vi "TDMS.SetMetadata.vi"(0 "Data":path, 2 "DUTs.AppVersion":string, 11 "error in (no error)":errorcluster, 13 "DUTs.BootVersion":string) -> (15 "error out":errorcluster)   [LabVIEW 2014, in "ParametericRoutines.lvlib"]
uses:
  ParametericRoutines.lvlib
  Constants.vi
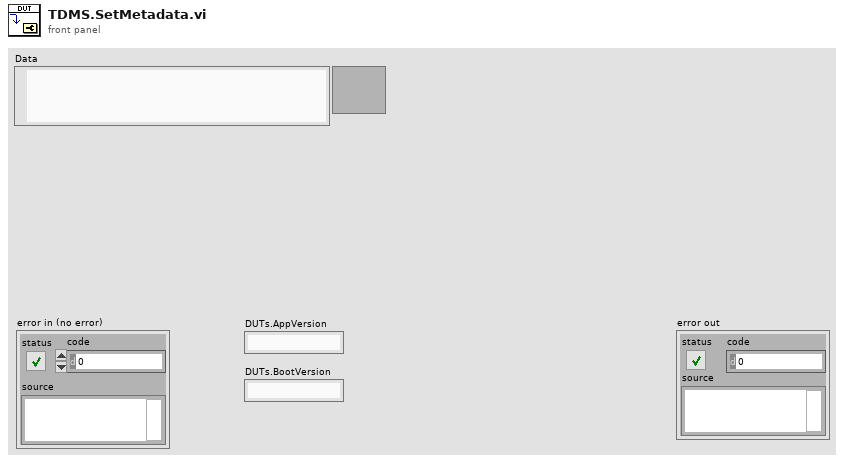
[diagram p1: front panel]
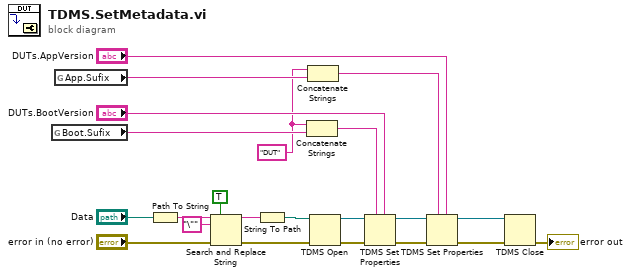
[diagram p0: block diagram]
diagram:
  w3 = "DUT" ("Boot.Sufix")
  n1 = global read "Constants.vi" "Boot.Sufix"() -> (w13:string)
  n2 = global read "Constants.vi" "App.Sufix"() -> (w14:string)
  n3 = Path To String(path="Data") -> (string=w21:string)
  n4 = Search and Replace String(replace all?=TRUE ("replace all? (F)"), input string=w21, search string="\"", error in="error in (no error)") -> (result string=w22:string, error out=w16:errorcluster)  [unwired: 4 in, 2 out]
  n5 = String To Path(string=w22) -> (path=w17:path)
  n6 = Concatenate Strings(w3, w13) -> (w7:string)
  n7 = Concatenate Strings(w3, w14) -> (w6:string)
  n8 = TDMS Open(8:w16, 11:w17) -> (0:w1:errorcluster, 3:w2:refnum<k34>)  [unwired: 5 in]
  n9 = TDMS Set Properties(5:"DUTs.BootVersion", 7:w7, 8:w1, 11:w2) -> (0:w8:errorcluster, 3:w9:refnum<k34>)  [unwired: 2 in, 2 out]
  n10 = TDMS Set Properties(5:"DUTs.AppVersion", 7:w6, 8:w8, 11:w9) -> (0:w12:errorcluster, 3:w11:refnum<k34>)  [unwired: 2 in, 2 out]
  n11 = TDMS Close(8:w12, 11:w11) -> (0:→"error out":errorcluster)  [unwired: 1 out]
